vi "Pulse Attribute, Get Results.vi"(5 "Labels":string[](array[string])=["Stim Amp (mA)", "Stim Pulse Width (us)", "Interphase Delay (us)", "Recvy Amp (mA)", "Recvy Pulse Width (us)", "Frequency (Hz)", "Period Jitter (us rms)"], 6 "error in":errorcluster, 9 "waveform":waveform(dbl)={"t0"=timestamp(3473168073.631 s since 1904-01-01), "dt"=1e-08, "Y"=[], "attributes"=variant("Average Size"=variant(dbl 15.0), "Frequency (Hz)"=variant(dbl 1998.0127546741205), "Interphase Delay (us)"=variant(dbl 15.772500000000003), "MD5[0]"=variant(dbl 3432209604.0), "MD5[1]"=variant(dbl 1216260660.0), "MD5[2]"=variant(dbl 1007192998.0), "MD5[3]"=variant(dbl 1264973305.0), "NSamp"=variant(dbl 400000.0), "Number of Samples"=variant(dbl 400000.0), "Process Timestamp"=variant(dbl 3475173434.5), "Recvy Amp (V)"=variant(dbl 2.6382379145344714), "Recvy Amp (mA)"=variant(dbl 5.276475829068943), "Recvy Duty Factor"=variant(dbl 0.024841948874633292), "Recvy Frequency (Hz)"=variant(dbl 1998.1571037522094), "Recvy Period (us)"=variant(dbl 500.4611489868164), "Recvy Pulse Width (us)"=variant(dbl 12.432430276870729), "Recvy Trigger (s)"=variant(dbl 0.00044008000000000003), "Resistance (ohms)"=variant(dbl 500.0), "Samp Freq (MHz)"=variant(dbl 100.0), "Sample Frequency (MHz)"=variant(dbl 100.0), "Stim Amp (V)"=variant(dbl -2.3035646134631413), "Stim Amp (mA)"=variant(dbl -4.607129226926283), "Stim Duty Factor"=variant(dbl 0.024124139362212305), "Stim Frequency (Hz)"=variant(dbl 1997.8684055960314), "Stim Period (us)"=variant(dbl 500.53346716880804), "Stim Pulse Width (us)"=variant(dbl 12.07493911743164), "Stim Trigger (s)"=variant(dbl 0.00041221), "dt (us)"=variant(dbl 0.01))}) -> (0 "error out":errorcluster, 3 "waveform dup":waveform(dbl)={"t0"=timestamp(0 s since 1904-01-01), "dt"=nan, "Y"=[]}, 4 "Results":T1[](array[typedef]) {"Value" format="%#.3f"})   [LabVIEW 2010]
doc: "This function extracts Test Results from the waveform attributes."
uses:
  Generic/Waveform Attribute/Waveform Attribute Cluster.ctl
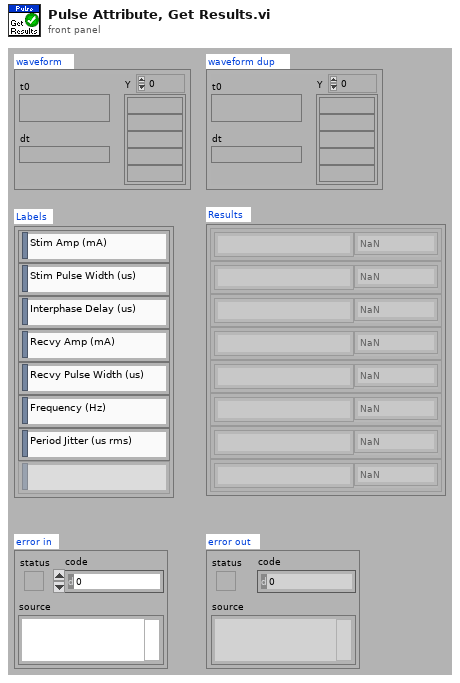
[diagram p1: front panel]
types:
  T1 = typedef "Waveform Attribute Cluster.ctl" = cluster{"Label":string, "Value":dbl}
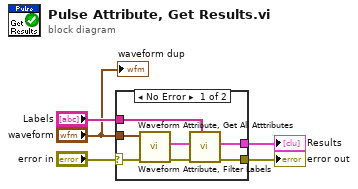
[diagram p0: block diagram]
diagram:
  n1 = case shown="No Error" "error in" {
    selector: "error in" -> [w10 w13]
    tunnel: "Labels" -> [w7 _]
    tunnel: [w9 w13] -> w3
    tunnel: [w8 _] -> w2
    tunnel: "waveform" -> [w6 _]
    frame No Error {
      n2 = call "Waveform Attribute, Get All Atttributes.vi"("error in"=w10, "waveform"=w6) -> ("error out"=w12:errorcluster, "all attributes"=w11:T1[])  [unwired: 5 in, 1 out]
      n3 = call "Waveform Attribute, Filter Labels.vi"("labels"=w7, "error in"=w12, "attributes"=w11) -> ("error out"=w9:errorcluster, "filtered results"=w8:T1[])  [unwired: 5 in]
    }
    frame Error {
    }
  }
  "Results" <- w2
  "error out" <- w3
  "waveform dup" <- "waveform"
